vi "Untitled 5 (SubVI).vi"(8 "error in (no error)":errorcluster, 9 "Cluster in":T1, 10 "Tree pics & devs in":string, 11 "TreeControl in":refnum<vi>) -> (0 "error out":errorcluster, 2 "Cluster out":T1, 3 "name":string)   [LabVIEW 2013, in "DataCreation.lvlib"]
uses:
  DataCreation.lvlib
  vis/SetupData2.ctl
  classes/Datastructure/Device/Device.lvclass
  classes/Datastructure/Image/img.lvclass
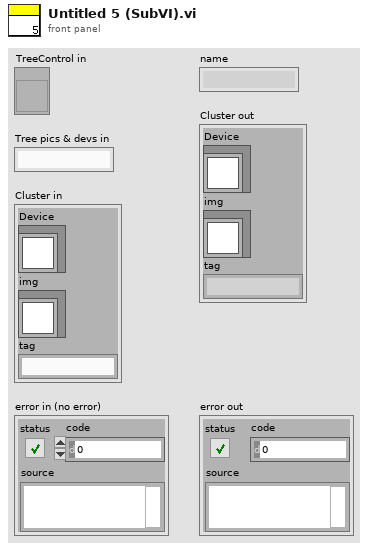
[diagram p1: front panel]
types:
  T1 = typedef "SetupData2.ctl" = cluster{"Device":refnum<class "Device.lvclass">, "img":refnum<class "img.lvclass">, "tag":string}
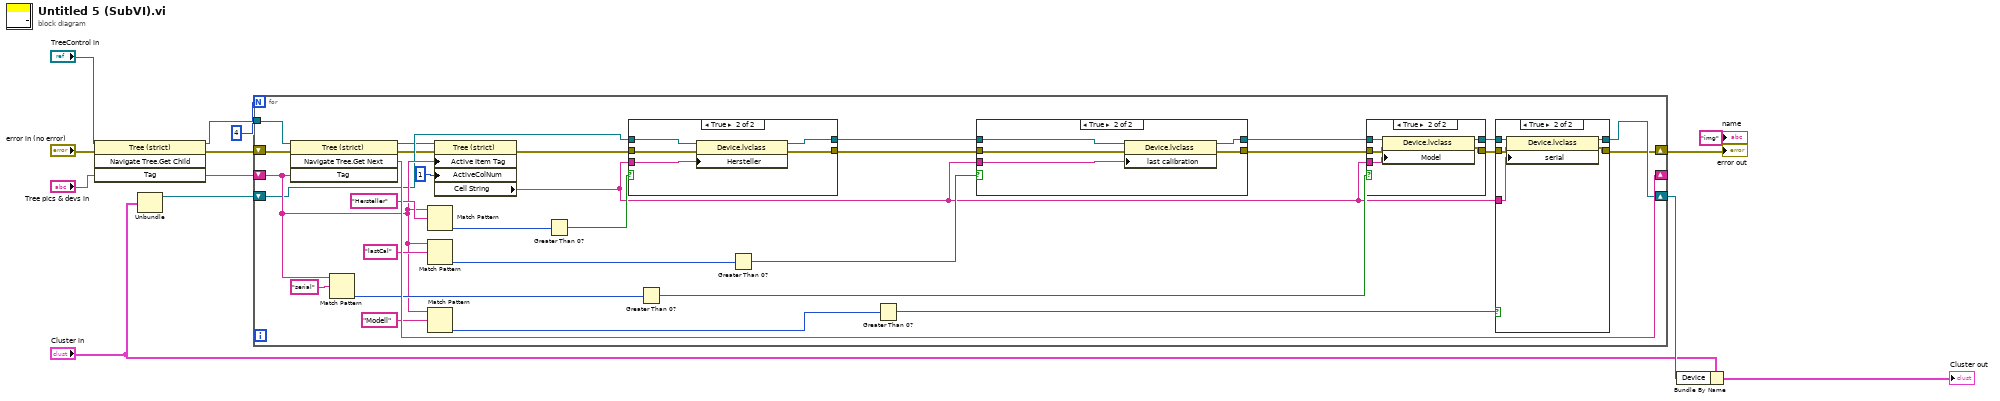
[diagram p0: block diagram]
diagram:
  n1 = invoke class="Tree (strict)" method="Navigate Tree.Get Child"(reference="TreeControl in", error in="error in (no error)", "Tag"="Tree pics & devs in") -> (reference out=w4:refnum<vi>, error out=w8:errorcluster)  [unwired: 1 in, 2 out]
  n2 = Unbundle("Cluster in") -> ("Device"=w9:refnum<class "Device.lvclass">)  [unwired: 2 out]
  n3 = for {
    N: 4 -> [_]
    tunnel: w4 -> [w21]
    shift-right: [w42] -> _
    shift-left: "Tree pics & devs in" -> [w31]
    shift-right: [w13] -> w11
    shift-left: w8 -> [w22]
    shift-right: [w23] -> w10
    shift-left: w9 -> [w27]
    n4 = invoke class="Tree (strict)" method="Navigate Tree.Get Next"(reference=w21, error in=w22, "Tag"=w31) -> (reference out=w14:refnum<vi>, error out=w18:errorcluster, "Navigate Tree:Get Next Item"=w42:string)  [unwired: 1 in, 1 out]
    n5 = Match Pattern(string=w31, regular expression="serial" ("Linker Zellen-String")) -> (offset past match=w36:i32)  [unwired: 1 in, 3 out]
    n6 = Match Pattern(string=w31, regular expression="Hersteller" ("Left Cell String")) -> (offset past match=w39:i32)  [unwired: 1 in, 3 out]
    n7 = Match Pattern(string=w31, regular expression="lastCal" ("Linker Zellen-String")) -> (offset past match=w37:i32)  [unwired: 1 in, 3 out]
    n8 = Match Pattern(string=w31, regular expression="Modell" ("Linker Zellen-String")) -> (offset past match=w35:i32)  [unwired: 1 in, 3 out]
    n9 = property class="Tree (strict)"(reference=w14, error in=w18, "Active Item Tag"=w31, "ActiveColNum"=1 ("Active Cell:Active Column Number")) -> (error out=w15:errorcluster, "Cell String"=w16:string)  [unwired: 1 out]
    n10 = Greater Than 0?(x=w39) -> (x > 0?=w40:bool)
    n11 = case shown="True" w40 {
      tunnel: w15 -> [w64 w70]
      tunnel: [w64 w69] -> w17
      tunnel: w27 -> [w65 w68]
      tunnel: [w65 w67] -> w26
      tunnel: w16 -> [_ w66]
      frame False {
      }
      frame True {
        n12 = property class="Device.lvclass"(reference=w68, error in=w70, "Hersteller"=w66) -> (reference out=w67:refnum<class "Device.lvclass">, error out=w69:errorcluster)
      }
    }
    n13 = Greater Than 0?(x=w36) -> (x > 0?=w29:bool)
    n14 = Greater Than 0?(x=w37) -> (x > 0?=w30:bool)
    n15 = Greater Than 0?(x=w35) -> (x > 0?=w28:bool)
    n16 = case shown="True" w30 {
      tunnel: w17 -> [w57 w63]
      tunnel: [w57 w62] -> w20
      tunnel: w26 -> [w58 w61]
      tunnel: [w58 w60] -> w25
      tunnel: w16 -> [_ w59]
      frame False {
      }
      frame True {
        n17 = property class="Device.lvclass"(reference=w61, error in=w63, "last calibration"=w59) -> (reference out=w60:refnum<class "Device.lvclass">, error out=w62:errorcluster)
      }
    }
    n18 = case shown="True" w29 {
      tunnel: w20 -> [w50 w56]
      tunnel: [w50 w55] -> w19
      tunnel: w25 -> [w51 w54]
      tunnel: [w51 w53] -> w24
      tunnel: w16 -> [_ w52]
      frame False {
      }
      frame True {
        n19 = property class="Device.lvclass"(reference=w54, error in=w56, "Model"=w52) -> (reference out=w53:refnum<class "Device.lvclass">, error out=w55:errorcluster)
      }
    }
    n20 = case shown="True" w28 {
      tunnel: w19 -> [w43 w49]
      tunnel: [w43 w48] -> w13
      tunnel: w24 -> [w44 w47]
      tunnel: [w44 w46] -> w23
      tunnel: w16 -> [_ w45]
      frame False {
      }
      frame True {
        n21 = property class="Device.lvclass"(reference=w47, error in=w49, "serial"=w45) -> (reference out=w46:refnum<class "Device.lvclass">, error out=w48:errorcluster)
      }
    }
  }
  "error out" <- w11
  n22 = Bundle By Name(cluster="Cluster in", "Device"=w10) -> (→"Cluster out":T1)
  "name" <- "img" ("name")
